vi "Ramp.vi"(8 "Negative Change":dbl, 9 "Positive Change":dbl, 10 "Prev Motor":dbl, 11 "Input":dbl) -> (1 "In range?":bool, 2 "Motor Output":dbl)   [LabVIEW 2014]
doc: "Fixes motor acceleration to a linear rate.\nInputs:\n AccelForward - Current forward acceleration limit\n AccelBackward - Current backward acceleration limit\n PrevMotor - The previous motor value\n Input - The new value to be given to the motor\nOutputs:\n Motor Output - The value to be sent to the motor\n In Range? - A boolean that tells you if the Input was within the specified range\nCode:\n The Input is coerced to be between the AccelForward + Prev Motor and Prev Motot - AccelBackward"
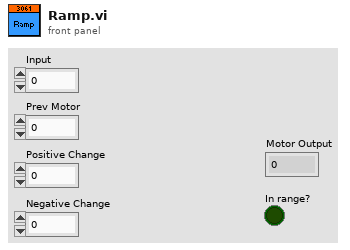
[diagram p1: front panel]
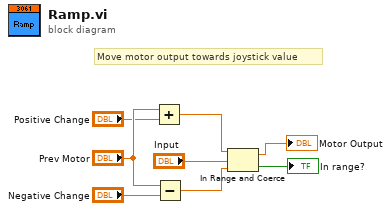
[diagram p0: block diagram]
diagram:
  # "Move motor output towards joystick value"
  n1 = Add(x="Prev Motor", y="Positive Change") -> (x+y=w5:dbl)
  n2 = Subtract(x="Prev Motor", y="Negative Change") -> (x-y=w4:dbl)
  n3 = In Range and Coerce(upper limit=w5, x="Input", lower limit=w4) -> (coerced(x)=→"Motor Output":dbl, In Range?=→"In range?":bool)
